vi "u8_to_sev_seg.vi"(1 "Numeric":u8 format="%x") -> (0 "Digit":T1)   [LabVIEW 2018]
uses:
  seven_seg_digit.ctl
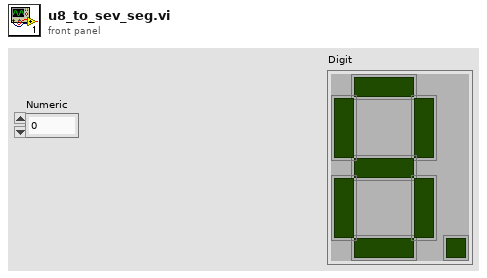
[diagram p1: front panel]
types:
  T1 = typedef "seven_seg_digit.ctl" = cluster{"DP":bool, "A":bool, "B":bool, "C":bool, "D":bool, "E":bool, "F":bool, "G":bool}
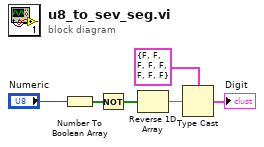
[diagram p0: block diagram]
diagram:
  n1 = Number To Boolean Array(number="Numeric") -> (Boolean array=w3:bool[])
  n2 = Not(x=w3) -> (.not. x?=w1:bool[])
  n3 = Reverse 1D Array(array=w1) -> (reversed array=w2:bool[])
  n4 = Type Cast(type=T1 {"DP"=FALSE, "A"=FALSE, "B"=FALSE, "C"=FALSE, "D"=FALSE, "E"=FALSE, "F"=FALSE, "G"=FALSE} ("Digit 2"), x=w2) -> (*(type *) &x=→"Digit":T1)
